vi "ReadingMyAttribute.vi"(0 "reference in":refnum<class "MyG#G3Templ.lvclass">, 5 "error in (no error)":errorcluster) -> (14 "reference out":refnum<class "MyG#G3Templ.lvclass">, 15 "MyAttribute":dbl, 19 "error out":errorcluster)   [LabVIEW 2020, in "MyG#G3Templ.lvclass"]
uses:
  MyG#G3Templ.lvclass
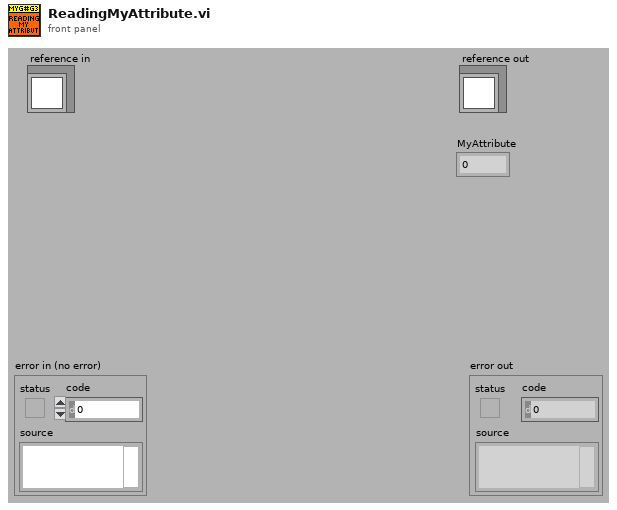
[diagram p1: front panel]
types:
  T1 = typedef "MyG#G3Templ.lvclass/ObjectAttributes.ctl" = cluster{"MyAttribute":dbl}
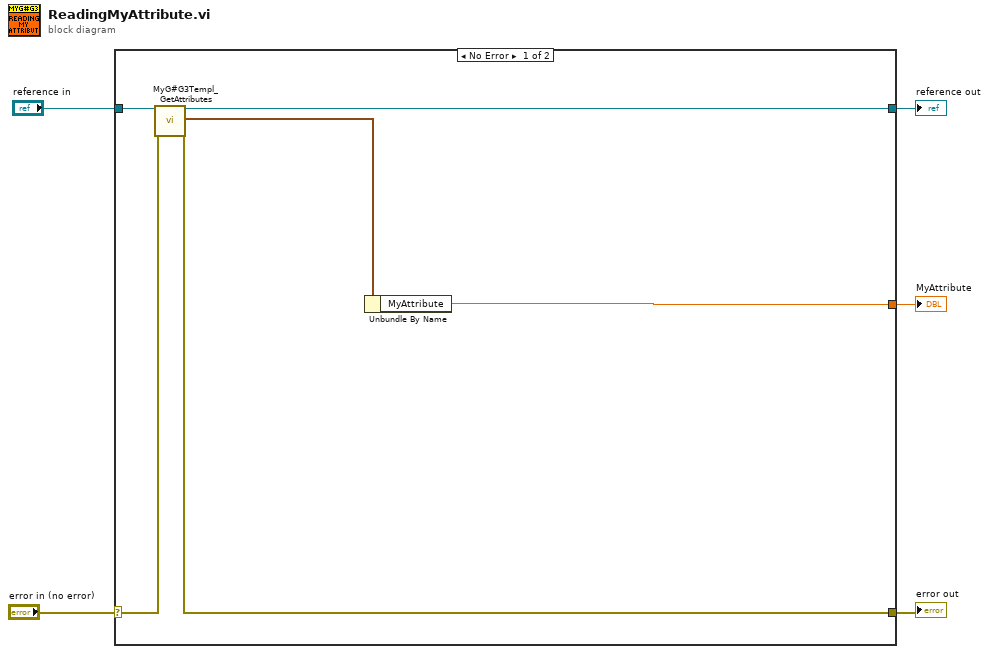
[diagram p0: block diagram]
diagram:
  n1 = case shown="No Error" "error in (no error)" {
    selector: "error in (no error)" -> [w11 w13]
    tunnel: [w9 w13] -> w4
    tunnel: [w7 w12] -> w2
    tunnel: "reference in" -> [w8 w12]
    tunnel: [w6 _] -> w1
    frame No Error {
      n2 = call "MyG#G3Templ_GetAttributes.vi"("reference in"=w8, "error in (no error)"=w11) -> ("reference out"=w7:refnum<class "MyG#G3Templ.lvclass">, "attributes"=w10:T1, "error out"=w9:errorcluster)  [unwired: 14 in, 1 out]
      n3 = Unbundle By Name(w10) -> ("MyAttribute"=w6:dbl)
    }
    frame Error {
    }
  }
  "error out" <- w4
  "reference out" <- w2
  "MyAttribute" <- w1
